vi "EditValue.vi"(8 "error in (no error)":errorcluster, 10 "Bounds":T1, 11 "Dropdown D Element in":refnum<class "String dropdown D Element.lvclass">) -> (0 "error out":errorcluster, 1 "Tabbed out?":bool, 2 "Value changed?":bool, 3 "Dropdown D Element out":refnum<class "String dropdown D Element.lvclass">)   [LabVIEW 2018, in "D Datagrid Library.lvlib" / "String dropdown D Element.lvclass"]
uses:
  String dropdown D Element.lvclass
  <vilib>/Utility/miscctls.llb/LVRectTypeDef.ctl
  String dropdown D Element.lvclass/String dropdown D Element.ctl
  Read value.vi
  Read Strings.vi
  Write value.vi
panel:
  in  "Listbox":i32(listbox)
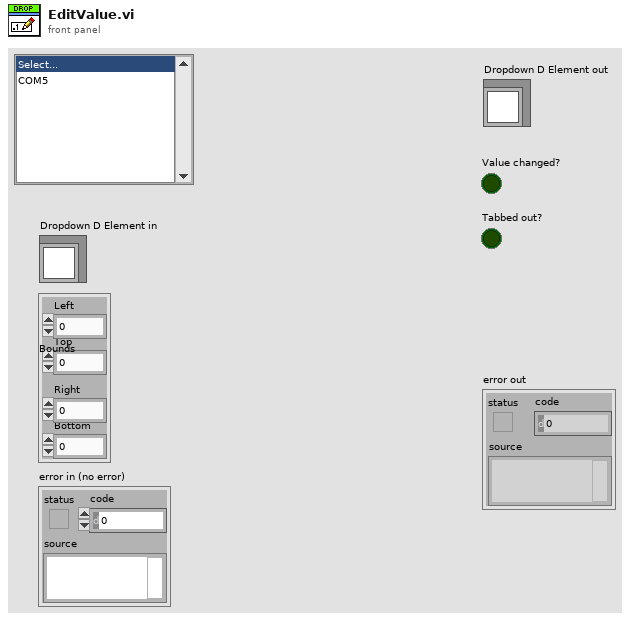
[diagram p1: front panel]
types:
  T1 = typedef "LVRectTypeDef.ctl" = cluster{"Left":i16, "Top":i16, "Right":i16, "Bottom":i16}
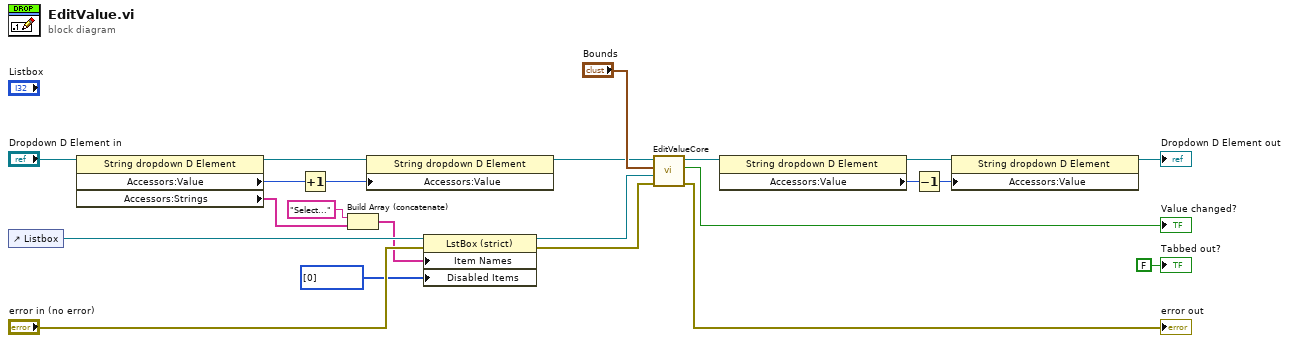
[diagram p0: block diagram]
diagram:
  n1 = control-ref of="Listbox"() -> (w16:refnum<vi>)
  n2 = property class="String dropdown D Element"(reference="Dropdown D Element in") -> (reference out=w7:refnum<class "String dropdown D Element.lvclass">, "Accessors:Value"=w6:i32, "Accessors:Strings"=w2:string[])  [unwired: 1 in, 1 out]
  n3 = Increment(x=w6) -> (x+1=w5:i32)
  n4 = Build Array (concatenate)("Select...", w2) -> (w3:string[])
  n5 = property class="String dropdown D Element"(reference=w7, "Accessors:Value"=w5) -> (reference out=w8:refnum<class "String dropdown D Element.lvclass">)  [unwired: 1 in, 1 out]
  n6 = property class="LstBox (strict)"(reference=w16, error in="error in (no error)", "Item Names"=w3, "Disabled Items"=i32[] [0]) -> (reference out=w22:refnum<vi>, error out=w17:errorcluster)
  n7 = call-dynamic "EditValueCore.vi"("error in (no error)"=w17, "Value field reference"=w22, "Bounds"="Bounds", "DatagridElement in"=w8) -> ("error out"=→"error out":errorcluster, "Value changed?"=→"Value changed?":bool, "DatagridElement out"=w11:refnum<class "String dropdown D Element.lvclass">)  [unwired: 4 in, 1 out]
  n8 = property class="String dropdown D Element"(reference=w11) -> (reference out=w14:refnum<class "String dropdown D Element.lvclass">, "Accessors:Value"=w13:i32)  [unwired: 1 in, 1 out]
  n9 = Decrement(x=w13) -> (x-1=w12:i32)
  n10 = property class="String dropdown D Element"(reference=w14, "Accessors:Value"=w12) -> (reference out=→"Dropdown D Element out":refnum<class "String dropdown D Element.lvclass">)  [unwired: 1 in, 1 out]
  "Tabbed out?" <- FALSE ("Tabbed out?")
